vi "solar_msg UE Create.vi"(8 "error in (no error)":errorcluster) -> (0 "error out":errorcluster, 3 "UserEvent":refnum<user-event>)   [LabVIEW 2018]
doc: "This creates a <b>User Event</b> reference."
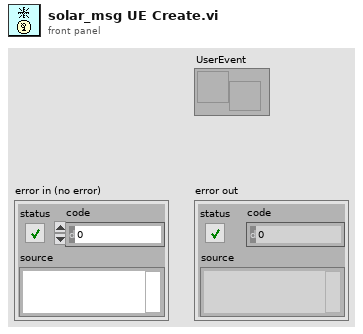
[diagram p1: front panel]
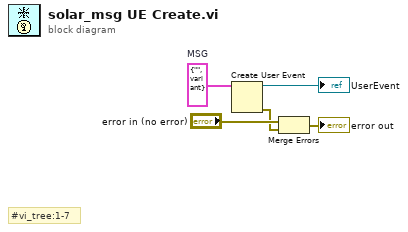
[diagram p0: block diagram]
diagram:
  w2 = cluster{"MSG":string, "DATA":variant} {"MSG"="", "DATA"=variant}  # MSG
  # "#vi_tree:1-7"
  n1 = Create User Event(user event datatype=w2) -> (user event=→"UserEvent":refnum<user-event>, error out=w3:errorcluster)  [unwired: 1 in]
  n2 = Merge Errors("error in (no error)", w3) -> (→"error out":errorcluster)
